vi "test.vi"() -> ()   [LabVIEW 2019]
uses:
  <vilib>/Platform/TimedLoop/XDataNode/timing_clust.ctl
  <vilib>/Platform/TimedLoop/XDataNode/nitl_modes.ctl
  <vilib>/Platform/TimedLoop/XDataNode/wakeup.ctl
  Downloads/WSCBOTV3 -20210128T063933Z-001/WSCBOTV3/WSCBOTV3_Toolkit/Sensor/LowLevel/IR_Chanel.ctl
  Downloads/WSCBOTV3 -20210128T063933Z-001/WSCBOTV3/WSCBOTV3_Toolkit/Sensor/LowLevel/InfraredRanging(Array).vi
  <vilib>/Platform/TimedLoop/XDataNode/XDataNode.xnode
  <vilib>/Platform/TimedLoop/XDataNode/XDNodeRunTimeDep.lvlib
panel:
  in  "Stop Button":bool
  out "Waveform Chart":T1(graph)
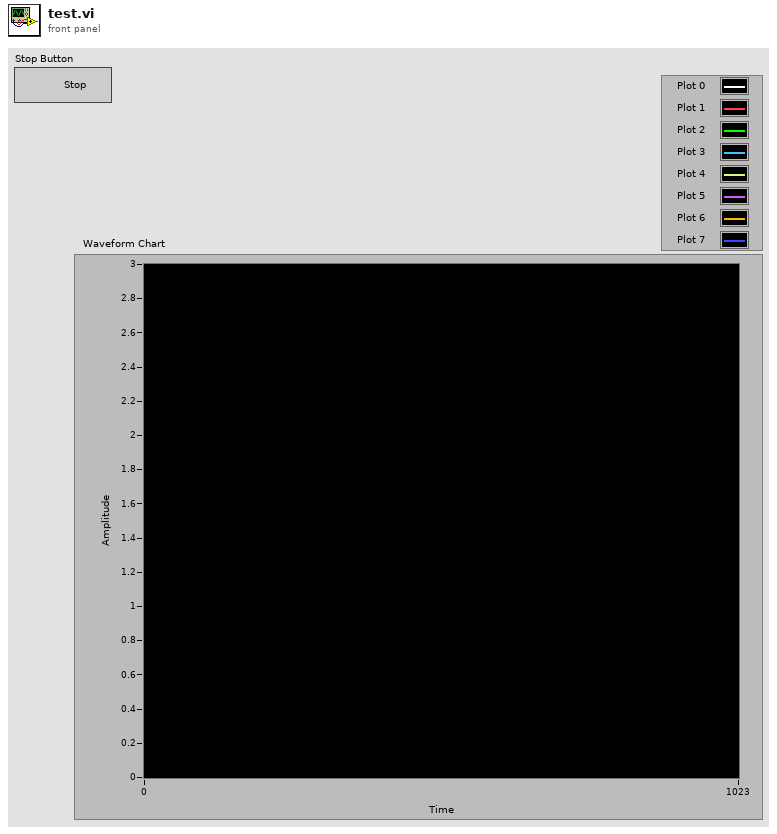
[diagram p1: front panel]
types:
  T1 = cluster{"Valtage[0]":dbl, "Valtage[1]":dbl, "Valtage[2]":dbl, "Valtage[3]":dbl, "Valtage[4]":dbl, "Valtage[5]":dbl, "Valtage[6]":dbl, "Valtage[7]":dbl, "Valtage[8]":dbl}
  T2 = typedef "XDNodeRunTimeDep.lvlib/timing_clust.ctl" = cluster{"Expected End [f-1]":u64, "Actual End [f-1]":u64, "Finished Late? [f-1]":bool, "Expected End [i-1]":u64, "Actual End [i-1]":u64, "Finished Late? [i-1]":bool, "Expected Start [i]":u64, "Actual Start [i]":u64, "Expected Start [f]":u64, "Actual Start [f]":u64, "Source Name":string, "Structure Name":string, "Period":i64, "Deadline":i64, "Offset":i64, "Start":i64, "Priority":i32, "Timeout":i32, "Mode":T3, "Wakeup Reason":T4, "Error":errorcluster, "Source Type":string, "Secondary Source Type":string, "Global End Time":u64, "Global Start Time":u64, "Frame Duration":u64, "Iteration Duration":u64, "Assigned CPU":i32, "I/O Scan Engine Mode":u32}
  T3 = typedef "XDNodeRunTimeDep.lvlib/nitl_modes.ctl" = enum32{"No Change", "Process missed periods, maintain original phase", "Discard missed periods, maintain original phase", "Process missed periods, ignore original phase", "Discard missed periods, ignore original phase"}
  T4 = typedef "XDNodeRunTimeDep.lvlib/wakeup.ctl" = enum32{"Normal", "Aborted", "Asynchronous wakeup", "Timing source error", "Timed loop error", "Timeout"}
  T5 = typedef "IR_Chanel.ctl" = enum16{"IR_LF", "IR_LB", "IR_BL", "IR_BR", "IR_RB", "IR_RF", "IR_FR", "IR_FL"}
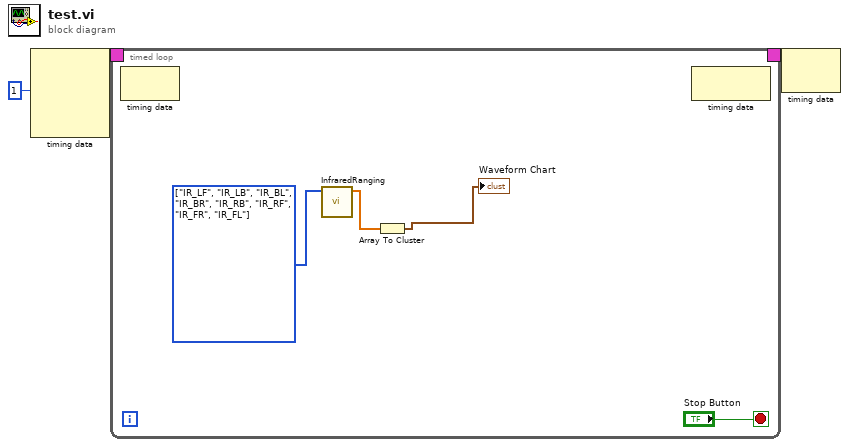
[diagram p0: block diagram]
diagram:
  n1 = node-c288(i64 1 ("Period")) -> (w3:T2)  [unwired: 3 in]
  n2 = timed-loop {
    timing: w3 -> [_]
    timing-out: [_] -> w2
    stop <- "Stop Button" stop-if-true
    w7 = T5[] [enum."IR_LF", enum."IR_LB", enum."IR_BL", enum."IR_BR", enum."IR_RB", enum."IR_RF", enum."IR_FR", enum."IR_FL"] items=["IR_LF", "IR_LB", "IR_BL", "IR_BR", "IR_RB", "IR_RF", "IR_FR", "IR_FL"] ("IR_Chanel")
    n3 = node-c288() -> ()  [unwired: 1 in, 1 out]
    n4 = call-poly "InfraredRanging.vi"("IR_Chanel"=w7) -> ("Valtage"=w6:dbl[])  [unwired: 9 in, 1 out]
    n5 = Array To Cluster(array=w6) -> (cluster=→"Waveform Chart":T1)
    n6 = node-c288() -> ()  [unwired: 1 in, 1 out]
  }
  n7 = node-c288(w2) -> ()  [unwired: 1 out]
